vi "Bump.vi"(8 "Error In":errorcluster, 11 "Parser In":refnum<class "Parser.lvclass">) -> (0 "Error Out":errorcluster, 2 "Done":bool, 3 "Parser Out":refnum<class "Parser.lvclass">)   [LabVIEW 2017, in "Mustache.lvlib" / "Parser.lvclass"]
uses:
  Parser.lvclass
  Parser.lvclass/Parser.ctl
  Readers/Public/Abstract/Abstract.lvclass
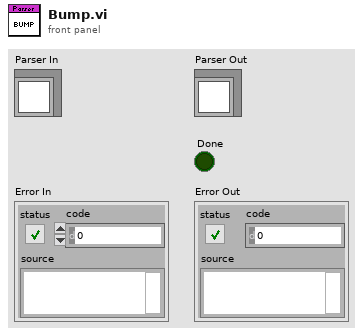
[diagram p1: front panel]
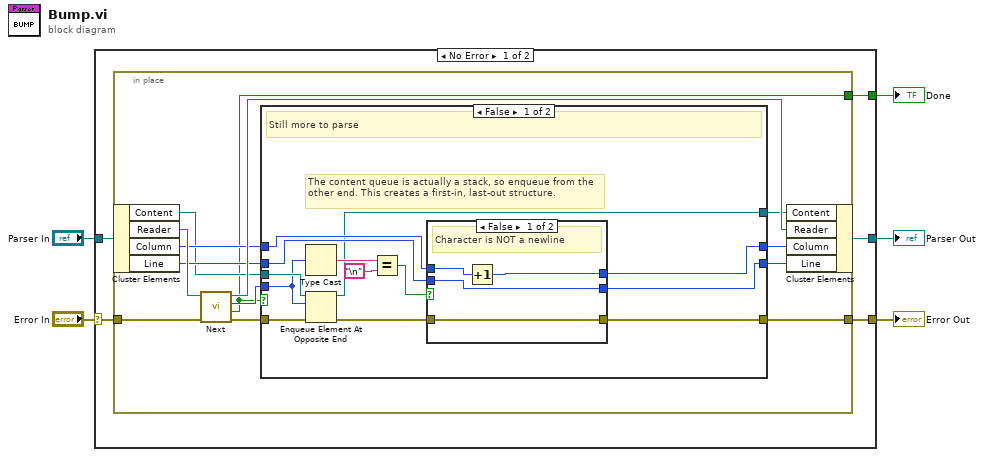
[diagram p0: block diagram]
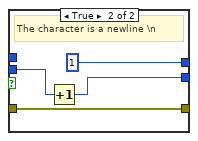
[diagram p2: hidden frame]
diagram:
  n1 = case shown="No Error" "Error In" {
    selector: "Error In" -> [w10 w50]
    tunnel: [w9 w50] -> w4
    tunnel: "Parser In" -> [w8 w49]
    tunnel: [w7 w49] -> w2
    tunnel: [w6 _] -> w1
    frame No Error {
      n2 = in-place {
        in-place-border: w10 -> [w23]
        in-place-border: [w19] -> w9
        in-place-border: [w11] -> w6
        n3 = in-place-cluster #1(w8) -> ("Content"=w13:refnum<queue>, "Reader"=w22:refnum<class "Abstract.lvclass">, "Column"=w18:u64, "Line"=w16:u64)
        n4 = call-dynamic "Next.vi"("Error In"=w23, "Reader In"=w22) -> ("Error Out"=w20:errorcluster, "Done"=w11:bool, "Character"=w14:u8, "Reader Out"=w21:refnum<class "Abstract.lvclass">)  [unwired: 6 in]
        n5 = case shown="False" w11 {
          tunnel: w20 -> [w27 w48]
          tunnel: [w36 w48] -> w19
          tunnel: w18 -> [w34 w47]
          tunnel: [w33 w47] -> w17
          tunnel: w16 -> [w32 w46]
          tunnel: [w31 w46] -> w15
          tunnel: w14 -> [w24 _]
          tunnel: w13 -> [w28 w45]
          tunnel: [w25 w45] -> w12
          frame False {
            # "The content queue is actually a stack, so enqueue from the other end. This creates a first-in, last-out structure."
            # "Still more to parse"
            n6 = Type Cast(x=w24) -> (*(type *) &x=w30:string)  [unwired: 1 in]
            n7 = Enqueue Element At Opposite End(queue=w28, element=w24, error in (no error)=w27) -> (queue out=w25:refnum<queue>, error out=w26:errorcluster)  [unwired: 1 in, 1 out]
            n8 = Equal?(x=w30, y="\n") -> (x = y?=w35:bool)
            n9 = case shown="False" w35 {
              tunnel: w26 -> [w38 w44]
              tunnel: [w38 w44] -> w36
              tunnel: w34 -> [w40 _]
              tunnel: [w39 u64 1 ("Column")] -> w33
              tunnel: w32 -> [w37 w42]
              tunnel: [w37 w41] -> w31
              frame False {
                # "Character is NOT a newline"
                n10 = Increment(x=w40) -> (x+1=w39:u64)
              }
              frame True {
                # "The character is a newline \\n"
                n11 = Increment(x=w42) -> (x+1=w41:u64)
              }
            }
          }
          frame True {
            # "End of Template (buffer, array, file, etc.)"
          }
        }
        n12 = in-place-cluster #1("Content"=w12, "Reader"=w21, "Column"=w17, "Line"=w15) -> (w7:refnum<class "Parser.lvclass">)
      }
    }
    frame Error {
    }
  }
  "Error Out" <- w4
  "Parser Out" <- w2
  "Done" <- w1
